vi "Destruct Data Block.vi"(8 "error in (no error)":errorcluster, 11 "Modbus Data Store in":refnum<class "MB Data Block.lvclass">) -> (0 "error out":errorcluster)   [LabVIEW 2018, in "MB PLC Client.lvlib" / "MB Data Block.lvclass"]
uses:
  MB Data Block.lvclass
  MB Data Block.lvclass/MB Data Block.ctl
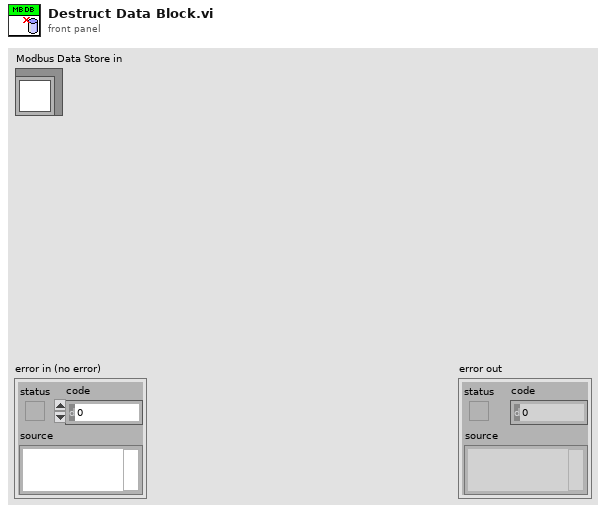
[diagram p1: front panel]
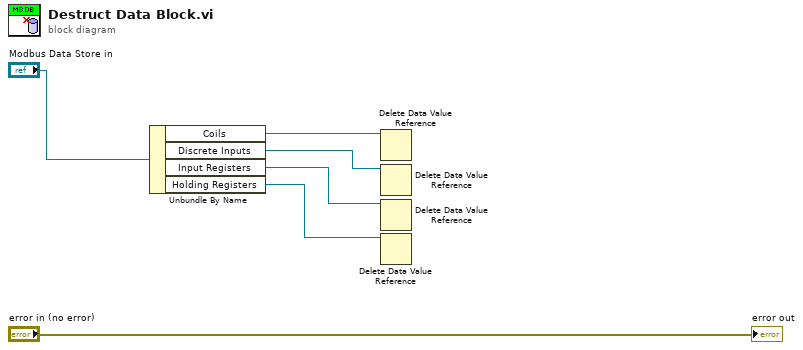
[diagram p0: block diagram]
diagram:
  n1 = Unbundle By Name("Modbus Data Store in") -> ("Coils"=w4:refnum<data-value>, "Discrete Inputs"=w3:refnum<data-value>, "Input Registers"=w2:refnum<data-value>, "Holding Registers"=w1:refnum<data-value>)
  n2 = Delete Data Value Reference(data value reference=w4) -> ()  [unwired: 1 in, 2 out]
  n3 = Delete Data Value Reference(data value reference=w3) -> ()  [unwired: 1 in, 2 out]
  n4 = Delete Data Value Reference(data value reference=w2) -> ()  [unwired: 1 in, 2 out]
  n5 = Delete Data Value Reference(data value reference=w1) -> ()  [unwired: 1 in, 2 out]
  "error out" <- "error in (no error)"
